vi "PH_gentec_M-Link.set Block Signal.vi"(0 "i ref in":refnum<vi>, 2 "VISA resource in":refnum<visa-resource-name>, 5 "error in":errorcluster) -> (14 "i ref out":refnum<vi>, 16 "VISA resource out":refnum<visa-resource-name>, 17 "Error":bool, 19 "error out":errorcluster)   [LabVIEW 2014, in "PH_gentec_M-Link.lvlib"]
doc: "This VI writes wanted Settings to the Device and checks the result."
uses:
  PH_gentec_M-Link.lvlib
  instr.lib/Gentec-M-Link/gentec-M-Link - Driver.lvlib
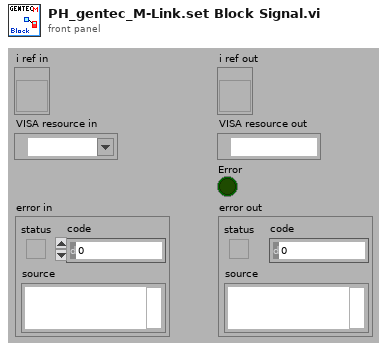
[diagram p1: front panel]
types:
  T1 = typedef "PH_gentec_M-Link.lvlib/PH_gentec_M-Link.i attribute.ctl" = cluster{"GUI References":cluster{"Wanted Head Settings":refnum<vi>, "Current Head Settings":refnum<vi>, "Set Auto Range":refnum<vi>, "Trigger Polarity":refnum<vi>, "Trigger Source":refnum<vi>, "Waveform Averages":refnum<vi>, "Continuous":refnum<vi>, "get one Value":refnum<vi>}, "Wanted Head Settings":T2, "Current Head Settings":T2}
  T2 = typedef "PH_gentec_M-Link.lvlib/PH_gentec_M-Link.Head Settings.ctl" = cluster{"Measurement Mode":T3, "Enable Anticipation":bool, "Set Auto Range":bool, "Block Signal":bool, "Set Head Attenuator":bool, "Enable SSE":bool, "Trigger Polarity":T4, "Trigger Source":T5, "Waveform Averages":T6, "Set Zero":i32, "Current Measurement":i32, "Start Data Flow":bool}
  T3 = typedef "gentec-M-Link - Driver.lvlib/gentec-M-Link.Measurement Mode.ctl" = u16
  T4 = typedef "gentec-M-Link - Driver.lvlib/gentec-M-Link.Trigger Polarity.ctl" = u16
  T5 = typedef "gentec-M-Link - Driver.lvlib/gentec-M-Link.Trigger Source.ctl" = u16
  T6 = typedef "gentec-M-Link - Driver.lvlib/gentec-M-Link.Waveform Averages.ctl" = u16
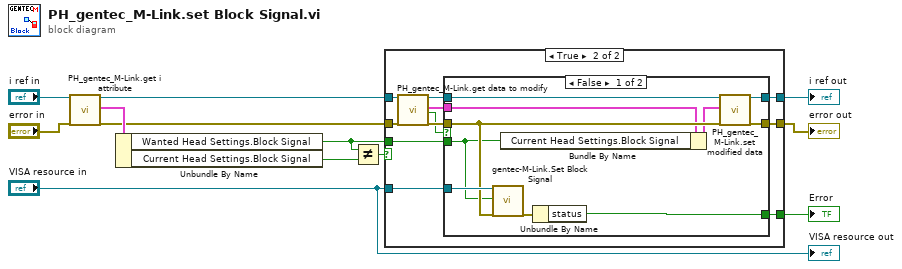
[diagram p0: block diagram]
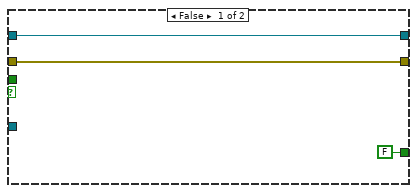
[diagram p2: hidden frame]
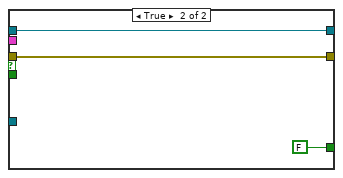
[diagram p3: hidden frame]
diagram:
  n1 = call "PH_gentec_M-Link.get i attribute.vi"("i ref in"="i ref in", "error in (no error)"="error in") -> ("i ref out"=w5:refnum<vi>, "i attribute"=w8:T1, "error out"=w7:errorcluster)  [unwired: 15 in]
  n2 = Unbundle By Name(w8) -> ("Wanted Head Settings.Block Signal"=w9:bool, "Current Head Settings.Block Signal"=w10:bool)
  n3 = Not Equal?(x=w9, y=w10) -> (x != y?=w1:bool)
  n4 = case shown="True" w1 {
    tunnel: [w14 w26] -> w12
    tunnel: [w15 w25] -> w11
    tunnel: w9 -> [_ w24]
    tunnel: w7 -> [w14 w19]
    tunnel: w5 -> [w15 w18]
    tunnel: "VISA resource in" -> [_ w17]
    tunnel: [FALSE w16] -> w2
    frame False {
    }
    frame True {
      n5 = call "PH_gentec_M-Link.get data to modify.vi"("i ref in"=w18, "error in (no error)"=w19) -> ("i ref out"=w22:refnum<vi>, "i attribute"=w21:T1, "timed out"=w20:bool, "error out"=w23:errorcluster)  [unwired: 14 in]
      n6 = case shown="False" w20 {
        tunnel: w17 -> [w35 _]
        tunnel: [w32 w39] -> w25
        tunnel: [w31 w38] -> w26
        tunnel: w23 -> [w34 w38]
        tunnel: w22 -> [w36 w39]
        tunnel: w21 -> [w30 _]
        tunnel: w24 -> [w28 _]
        tunnel: [w29 FALSE ("status")] -> w16
        frame False {
          n7 = call "gentec-M-Link.Set Block Signal.vi"("VISA resource In"=w35, "Block Signal"=w28, "error in (no error)"=w34) -> ("error out"=w27:errorcluster)  [unwired: 15 in, 1 out]
          n8 = Bundle By Name(cluster=w30, "Current Head Settings.Block Signal"=w28) -> (w33:T1)
          n9 = Unbundle By Name(w27) -> ("status"=w29:bool)
          n10 = call "PH_gentec_M-Link.set modified data.vi"("i ref in"=w36, "i attribute"=w33, "error in (no error)"=w34) -> ("i ref out"=w32:refnum<vi>, "error out"=w31:errorcluster)  [unwired: 15 in]
        }
        frame True {
        }
      }
    }
  }
  "error out" <- w12
  "i ref out" <- w11
  "Error" <- w2
  "VISA resource out" <- "VISA resource in"
